vi "Send 1 Scan multi-channel.vi"(0 "Connection ID in":refnum<k5>, 5 "Channel":T2[](array[typedef]), 11 "error in (no error)":errorcluster) -> (3 "Out of Range":bool[](array[boolean]), 4 "Connection ID out":refnum<k5>, 6 "voltage data":sgl[](array[numeric]) format="%.5f", 8 "Scaled data":sgl[](array[numeric]) format="%.2f", 10 "Sensor cluster":T1[](array[typedef]) {"scaled" format="%.2f"; "voltage" format="%.2f"}, 12 "units":string[](array[string]), 14 "time (s)":dbl format="%<%X\n%x>T", 15 "error out":errorcluster)   [LabVIEW 2015]
uses:
  calibration/global scale array.vi
  DataServer/data send.ctl
  DAQ configuration/channel identifier.ctl
  DataServer/command cluster.ctl
  DataServer/command.ctl
  DAQ configuration/sensor cluster.ctl
panel:
  in  "TCP read":u32=5000
  in  "TCP write":u32=1000
  in  "data":T3 {"seconds since 1904" format="%.2f"; "voltage data" format="%.4f"}
  out "data out":T4 {"arbitrary time (s)" format="%.2f"; "voltage data" format="%.5f"}
  in  "command interface":T5={"command"=enum."Idle", "start time (ms)"=0, "Channel Indices"=[], "Scans per Sample"=1} {"Scans per Sample" min=1}
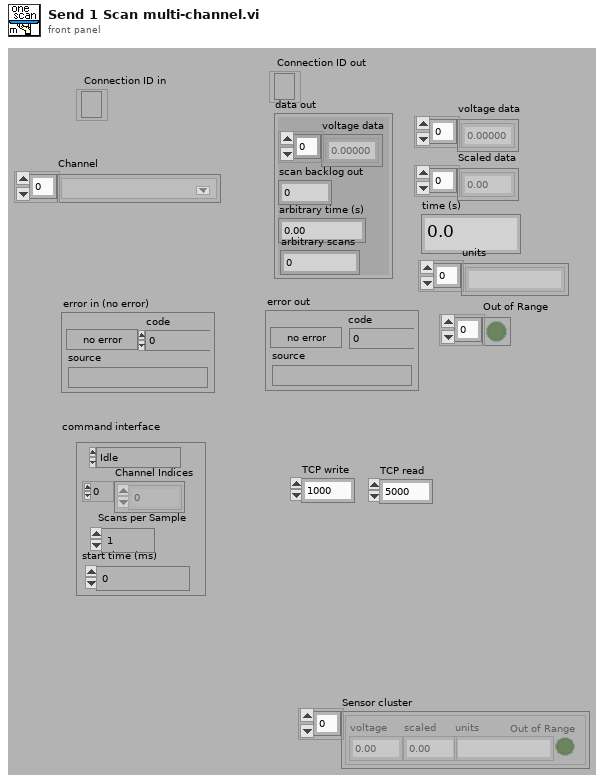
[diagram p1: front panel]
types:
  T1 = typedef "sensor cluster.ctl" = cluster{"voltage":sgl, "scaled":sgl, "units":string, "Out of Range":bool}
  T2 = typedef "channel identifier.ctl" = u16
  T3 = typedef "data send.ctl" = cluster{"voltage data":sgl[], "scan backlog":u32, "seconds since 1904":dbl, "arbitrary scans":i32}
  T4 = cluster{"voltage data":sgl[], "scan backlog out":u32, "arbitrary time (s)":dbl, "arbitrary scans":i32}
  T5 = typedef "command cluster.ctl" = cluster{"command":T6, "start time (ms)":u32, "Channel Indices":i32[], "Scans per Sample":i32}
  T6 = typedef "command.ctl" = enum16{"Idle", "Send Data", "Send 1 Scan", "Logoff"}
  T7 = enum16{"Standard", "Buffered", "CRLF", "Immediate"}
  T8 = enum16{"Idle", "Send Data", "Send 1 Scan", "Logoff"}
  T9 = typedef "calib array.ctl" = T10[]
  T10 = typedef "conversion.ctl" = cluster{"conversion matrix":sgl[][], "units":string, "name":string, "scale type":T11, "offset (volts)":dbl, "second channel":i8, "correspondence table":T12, "offset (physical units)":dbl, "pH scale":T13, "D.O.":T14, "Photometer data":T15}
  T11 = typedef "scale type.ctl" = enum16{"Volts", "Polynomial", "Correspondence Table", "pH", "Dissolved Oxygen", "Quadratic", "Photometer"}
  T12 = typedef "correspondence table.ctl" = cluster{"physical units":dbl, "volts":dbl}[]
  T13 = typedef "pH scale.ctl" = cluster{"Buffers":cluster{"Buffer":dbl, "Calibrated":bool, "V/T":dbl}[], "Temperature":dbl}
  T14 = typedef "DO scale.ctl" = cluster{"Temperature":dbl, "K":dbl, "barometric pressure":dbl}
  T15 = typedef "Photometer calibration data.ctl" = cluster{"Dark Voltage":dbl, "Blank Voltage":dbl, "Standards":cluster{"Concentration":dbl, "Voltage":dbl}[]}
  T16 = cluster{"voltage":sgl, sgl, "units":string, "Out of Range":bool}[]
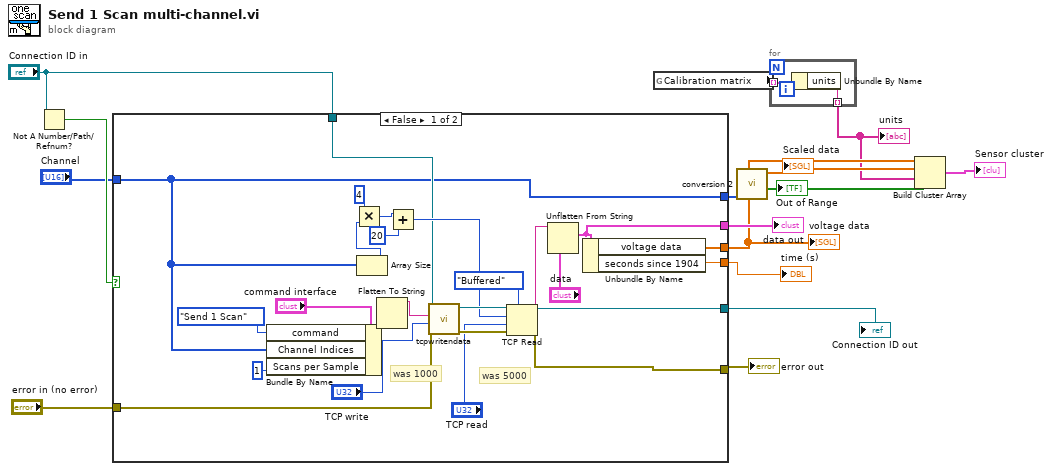
[diagram p0: block diagram]
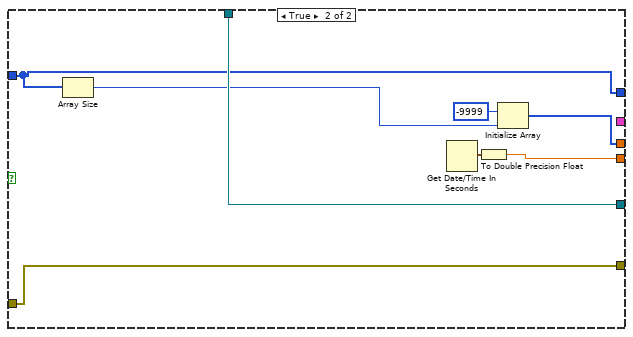
[diagram p2: hidden frame]
diagram:
  n1 = Not A Number/Path/Refnum?(number/path/refnum="Connection ID in") -> (NaN/Path/Refnum?=w4:bool)
  n2 = case shown="False" w4 {
    tunnel: [w33 _] -> w15
    tunnel: [w30 w48] -> w14
    tunnel: [w29 w45] -> w13
    tunnel: [w28 w47] -> w12
    tunnel: [w22 w42] -> w11
    tunnel: "Connection ID in" -> [w18 w48]
    tunnel: [w16 w41] -> w5
    tunnel: "error in (no error)" -> [w17 w47]
    tunnel: "Channel" -> [w16 w41]
    frame False {
      # "was 1000"
      # "was 5000"
      n3 = Bundle By Name(cluster="command interface", "command"=T8."Send 1 Scan", "Channel Indices"=w16, "Scans per Sample"=1) -> (w38:T5)
      n4 = Array Size(array=w16) -> (size(s)=w21:i32)
      n5 = Multiply(x=4, y=w21) -> (x*y=w25:i32)
      n6 = Flatten To String(anything=w38) -> (data string=w40:string)  [unwired: 3 in, 2 out]
      n7 = Add(x=w25, y=20) -> (x+y=w23:i32)
      n8 = call "tcpwritendata.vi"("error in (no error)"=w17, "timeout ms (25000)"="TCP write", "data in"=w40, "refnum in"=w18) -> ("error out"=w31:errorcluster, "refnum out"=w32:refnum<k5>)  [unwired: 5 in, 1 out]
      n9 = TCP Read(connection ID=w32, bytes to read=w23, error in (no error)=w31, 7:T7."Buffered" ("mode (standard)"), 9:"TCP read") -> (connection ID out=w30:refnum<k5>, data out=w34:string, error out=w28:errorcluster)
      n10 = Unflatten From String(type="data", binary string=w34) -> (value=w33:T3)  [unwired: 3 in, 2 out]
      n11 = Unbundle By Name(w33) -> ("voltage data"=w22:sgl[], "seconds since 1904"=w29:dbl)
    }
    frame True {
      n12 = Array Size(array=w41) -> (size(s)=w44:i32)
      n13 = Get Date/Time In Seconds() -> (seconds since 1Jan1904=w46:timestamp)
      n14 = To Double Precision Float(number=w46) -> (double precision float=w45:dbl)
      n15 = Initialize Array(-9999 ("element"), w44) -> (w42:i32[])
    }
  }
  "Connection ID out" <- w14
  "error out" <- w12
  "data out" <- w15
  "time (s)" <- w13
  "voltage data" <- w11
  n16 = global read "global scale array.vi" "Calibration matrix"() -> (w7:T9)
  n17 = call "conversion 2.vi"(8:w5, "raw Data"=w11) -> ("Out of Range"=w9:bool[], "calibrated data"=w10:sgl[])  [unwired: 7 in, 1 out]
  "Scaled data" <- w10
  "Out of Range" <- w9
  n18 = for {
    tunnel: w7 -> [w50] mode=indexing
    tunnel: [w49] -> w6 mode=indexing
    n19 = Unbundle By Name(w50) -> ("units"=w49:string)
  }
  "units" <- w6
  n20 = Build Cluster Array(w11, w10, w6, w9) -> (→"Sensor cluster":T16)
